vi "FTW-JSON-Object-GetElements-DBL.vi"(0 "JSON Object":refnum<class "FTW-JSON.lvclass">, 5 "Keys":string[](array[string]), 11 "error in":errorcluster) -> (4 "JSON Object out":refnum<class "FTW-JSON.lvclass">, 6 "Values":dbl[](array[numeric]), 8 "All Found?":bool, 10 "Which Found?":bool[](array[boolean]), 15 "error out":errorcluster)   [LabVIEW 2013, in "FTW-JSON.lvclass"]
uses:
  FTW-JSON.lvclass
panel:
  # "Inputs"
  # "Outputs"
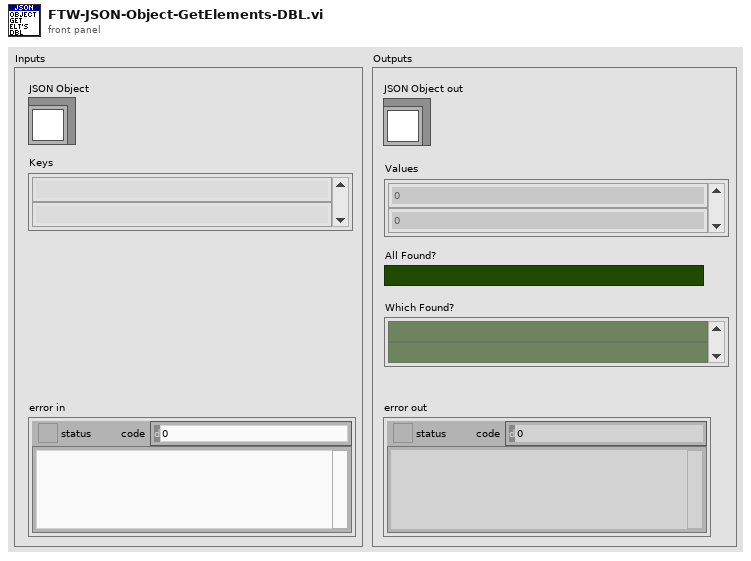
[diagram p1: front panel]
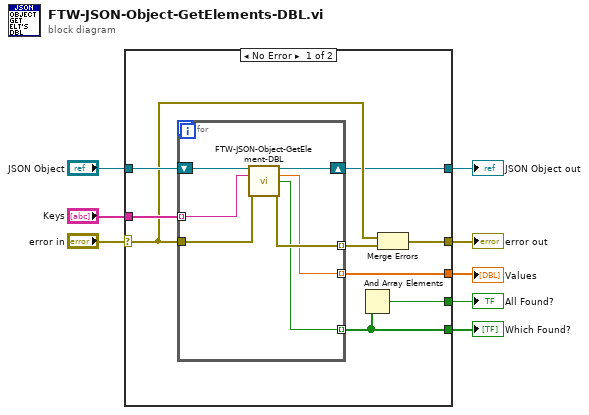
[diagram p0: block diagram]
diagram:
  n1 = case shown="No Error" "error in" {
    selector: "error in" -> [w13 w26]
    tunnel: [w17 w26] -> w8
    tunnel: [w10 w25] -> w6
    tunnel: "JSON Object" -> [w15 w25]
    tunnel: "Keys" -> [w14 _]
    tunnel: [w11 _] -> w3
    tunnel: [w16 _] -> w2
    tunnel: [w9 _] -> w1
    frame No Error {
      n2 = for {
        shift-right: [w21] -> w10
        shift-left: w15 -> [w24]
        tunnel: w14 -> [w23] mode=indexing
        tunnel: w13 -> [w22]
        tunnel: [w20] -> w12 mode=indexing
        tunnel: [w19] -> w11 mode=indexing
        tunnel: [w18] -> w9 mode=indexing
        n3 = call "FTW-JSON-Object-GetElement-DBL.vi"("JSON Object"=w24, "Key"=w23, "error in"=w22) -> ("JSON Object out"=w21:refnum<class "FTW-JSON.lvclass">, "Value"=w19:dbl, "Found?"=w18:bool, "error out"=w20:errorcluster)  [unwired: 9 in]
      }
      n4 = And Array Elements(Boolean array=w9) -> (logical AND=w16:bool)
      n5 = Merge Errors(w13, w12) -> (w17:errorcluster)
    }
    frame Error {
    }
  }
  "error out" <- w8
  "JSON Object out" <- w6
  "Values" <- w3
  "All Found?" <- w2
  "Which Found?" <- w1
